vi "Filter Path Name.vi"(0 "file or directory paths":path, 7 "filter for":T1, 11 "error in":errorcluster) -> (4 "matched file paths":path, 8 "matched":bool, 15 "error out":errorcluster)   [LabVIEW 2019, in "MD Generator.lvlib"]
uses:
  MD Generator.lvlib
  Filter.ctl
  <vilib>/regexp/Match Regular Expression.xnode
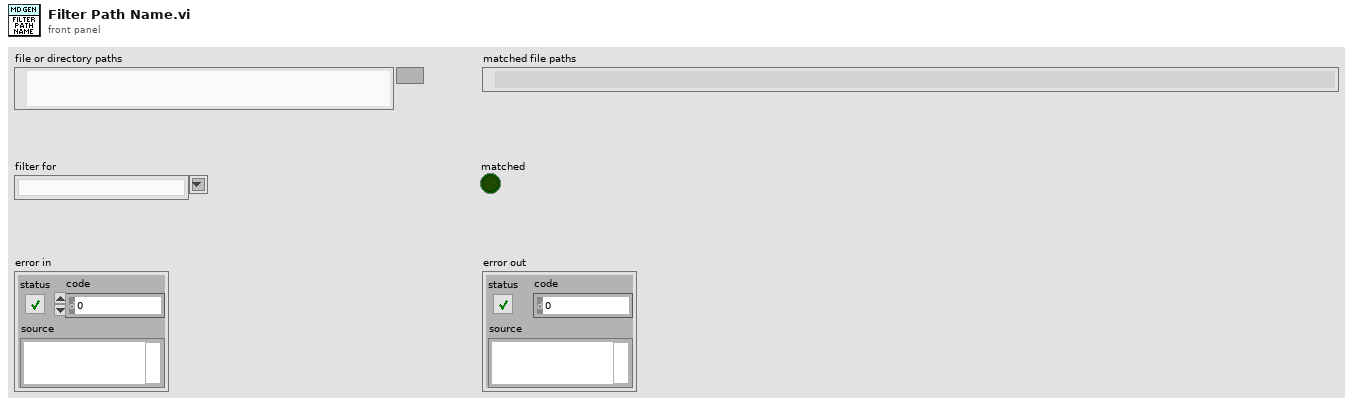
[diagram p1: front panel]
types:
  T1 = typedef "MD Generator.lvlib/Filter.ctl" = string
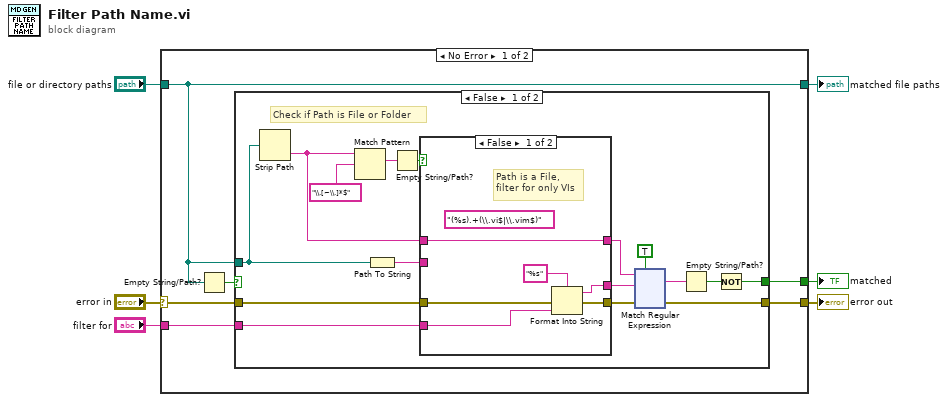
[diagram p0: block diagram]
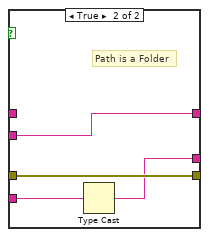
[diagram p2: hidden frame]
diagram:
  n1 = case shown="No Error" "error in" {
    selector: "error in" -> [w9 w155]
    tunnel: "file or directory paths" -> [w12 w154]
    tunnel: [w12 w154] -> w5
    tunnel: "filter for" -> [w11 _]
    tunnel: [w10 w155] -> w3
    tunnel: [w7 _] -> w1
    frame No Error {
      n2 = Empty String/Path?(string/path=w12) -> (empty?=w8:bool)
      n3 = case shown="False" w8 {
        tunnel: w11 -> [w17 _]
        tunnel: [w28 _] -> w7
        tunnel: [w24 w153] -> w10
        tunnel: w9 -> [w18 w153]
        tunnel: w12 -> [w23 _]
        frame False {
          # "Check if Path is File or Folder"
          n4 = Strip Path(path=w23) -> (name=w16:string)  [unwired: 1 out]
          n5 = Match Pattern(string=w16, regular expression="\\.[~\\.]*$") -> (match substring=w21:string)  [unwired: 4 out]
          n6 = Path To String(path=w23) -> (string=w14:string)
          n7 = Empty String/Path?(string/path=w21) -> (empty?=w13:bool)
          n8 = case shown="False" w13 {
            tunnel: [w29 w35] -> w20
            tunnel: [w34 w36] -> w19
            tunnel: w18 -> [w33 w36]
            tunnel: w17 -> [w31 w37]
            tunnel: w16 -> [w30 _]
            tunnel: [w30 w38] -> w15
            tunnel: w14 -> [_ w38]
            frame False {
              (unwired) "(%s).+(\\.vi$|\\.vim$)" ("format string")
              # "Path is a File,\nfilter for only VIs"
              n9 = Format Into String(format string="%s", error in=w33, w31) -> (resulting string=w29:string, error out=w34:errorcluster)  [unwired: 1 in]
            }
            frame True {
              # "Path is a Folder"
              n10 = Type Cast(x=w37) -> (*(type *) &x=w35:string)  [unwired: 1 in]
            }
          }
          n11 = xnode "Match Regular Expression"("input string"=w15, "regular expression"=w20, "error in"=w19, "ignore case? (F)"=TRUE) -> ("whole match"=w26:string, "error out"=w24:errorcluster)  [unwired: 2 in, 3 out]
          n12 = Empty String/Path?(string/path=w26) -> (empty?=w27:bool)
          n13 = Not(x=w27) -> (.not. x?=w28:bool)
        }
        frame True {
          # "Empty Path Do Not Propgate"
        }
      }
    }
    frame Error {
    }
  }
  "matched file paths" <- w5
  "error out" <- w3
  "matched" <- w1
